vi "VersionStrings.GetTypePalettePath.vi"(1 "Workspace Path":string) -> (0 "NI_VeristandTypes.ini File Path":string)   [LabVIEW 2014, in "VeriStand Steps Version Mutation.lvlib"]
uses:
  VeriStand Steps Version Mutation.lvlib
  Types/Constants.vi
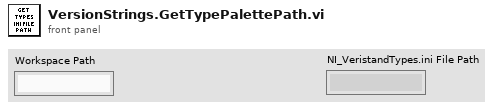
[diagram p1: front panel]
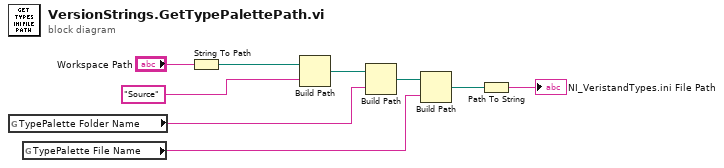
[diagram p0: block diagram]
diagram:
  n1 = global read "Constants.vi" "TypePalette Folder Name"() -> (w2:string)
  n2 = global read "Constants.vi" "TypePalette File Name"() -> (w1:string)
  n3 = String To Path(string="Workspace Path") -> (path=w5:path)
  n4 = Build Path(base path=w5, name or relative path="Source") -> (appended path=w9:path)
  n5 = Build Path(base path=w9, name or relative path=w2) -> (appended path=w7:path)
  n6 = Build Path(base path=w7, name or relative path=w1) -> (appended path=w8:path)
  n7 = Path To String(path=w8) -> (string=→"NI_VeristandTypes.ini File Path":string)
